vi "Error.GetError.vi"(11 "Msg":u8[](array[numeric])) -> (3 "error out":errorcluster)   [LabVIEW 2024, in "VS Plugin Inline Async API.lvlib"]
uses:
  VS Plugin Inline Async API.lvlib
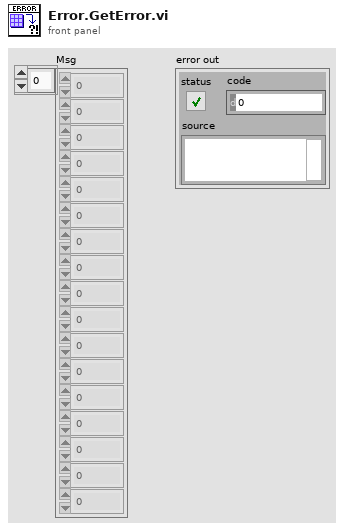
[diagram p1: front panel]
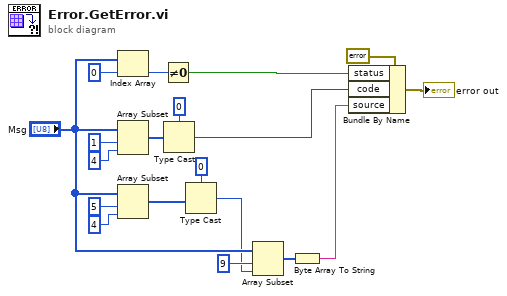
[diagram p0: block diagram]
diagram:
  n1 = Index Array(array="Msg", index=0) -> (element=w4:u8)
  n2 = Array Subset(array="Msg", index=1, length=4) -> (w9:u8[])
  n3 = Array Subset(array="Msg", index=5, length=4) -> (w10:u8[])
  n4 = Not Equal To 0?(x=w4) -> (x != 0?=w3:bool)
  n5 = Type Cast(type=0 ("code"), x=w9) -> (*(type *) &x=w2:i32)
  n6 = Type Cast(type=0 ("length"), x=w10) -> (*(type *) &x=w6:i32)
  n7 = Array Subset(array="Msg", index=9, length=w6) -> (w5:u8[])
  n8 = Byte Array To String(unsigned byte array=w5) -> (string=w1:string)
  n9 = Bundle By Name(cluster=errorcluster {"status"=FALSE, "code"=0, "source"=""} ("error in"), "status"=w3, "code"=w2, "source"=w1) -> (→"error out":errorcluster)
